vi "WriteTDMSTest1.vi"() -> ()   [LabVIEW 2016]
panel:
  out "Experiment Description 2":T1={"Sample Description"={"sample name"="SA01234.A", "device"="SA01234.A.20180713", "user"="patrick", "project"="graphene", "description"="sketch SET", "sample GUID"="3EAEE46B-2F5E-4712-8AE3-C241FD138412"}, "Experiment Description"={"folder name"="G:\\data\\graphene\\SA01234.A.20180713", "user description"="sweep Vsg as a function of B", "experiment GUID"="30E3DD13-C39C-4090-BB9A-3764BBD20948", "loop info (?)"=""}, "Krohn-Hite"={"Krohn-Hite Channel Array"=[{"channel"="Channel 1", "input config"="Differential", "gain"=100, "shunt resistor"=50, "input coupling"="", "filter"=""}, {"channel"="Channel 2", "input config"="Differential", "gain"=10, "shunt resistor"=50, "input coupling"="", "filter"=""}, {"channel"="Channel 3", "input config"="SE+ (-gnd)", "gain"=10, "shunt resistor"=0, "input coupling"="", "filter"=""}, {"channel"="Channel 4", "input config"="SE+ (-gnd)", "gain"=10, "shunt resistor"=0, "input coupling"="", "filter"=""}, {"channel"="Channel 5", "input config"="SE+ (-gnd)", "gain"=10, "shunt resistor"=0, "input coupling"="", "filter"=""}]}, "Lockin"={"Lockin AO"={"Lockin AO Channel Array"=[{"name"="0", "amplitude"=0.0, "DC offset"=0.0, "frequency"=13.0, "phase"=0.0, "function"="Sine"}, {"name"="1", "amplitude"=0.0, "DC offset"=0.0, "frequency"=13.0, "phase"=0.0, "function"="Sine"}, {"name"="2", "amplitude"=0.0, "DC offset"=0.0, "frequency"=13.0, "phase"=0.0, "function"="Sine"}, {"name"="3", "amplitude"=0.0, "DC offset"=0.0, "frequency"=13.0, "phase"=0.0, "function"="Sine"}, {"name"="4", "amplitude"=0.0, "DC offset"=0.0, "frequency"=13.0, "phase"=0.0, "function"="Sine"}, {"name"="5", "amplitude"=0.0, "DC offset"=0.0, "frequency"=13.0, "phase"=0.0, "function"="Sine"}, {"name"="6", "amplitude"=0.0, "DC offset"=0.0, "frequency"=13.0, "phase"=0.0, "function"="Sine"}, {"name"="7", "amplitude"=0.0, "DC offset"=0.0, "frequency"=13.0, "phase"=0.0, "function"="Sine"}]}, "Lockin AI"={"Lockin AI Array"=[{"KH Channel"="Channel 1", "AI Channel"="0"}, {"KH Channel"="Channel 2", "AI Channel"="1"}, {"KH Channel"="Channel 3", "AI Channel"="2"}, {"KH Channel"="Channel 4", "AI Channel"="3"}, {"KH Channel"="Channel 5", "AI Channel"="4"}]}, "Lockin REF"={"Lockin REF Array"=[{"frequency"=13.0, "phase"=0.0}]}}}
  out "date/time string":string="2018-10-02--21-17-20"
  out "current time":timestamp=timestamp(3621359841.3756013 s since 1904-01-01)
  in  "file path":path=path "C:/Users/Patrick/Desktop/TEST/TEST.tdms"
  in  "stop":bool
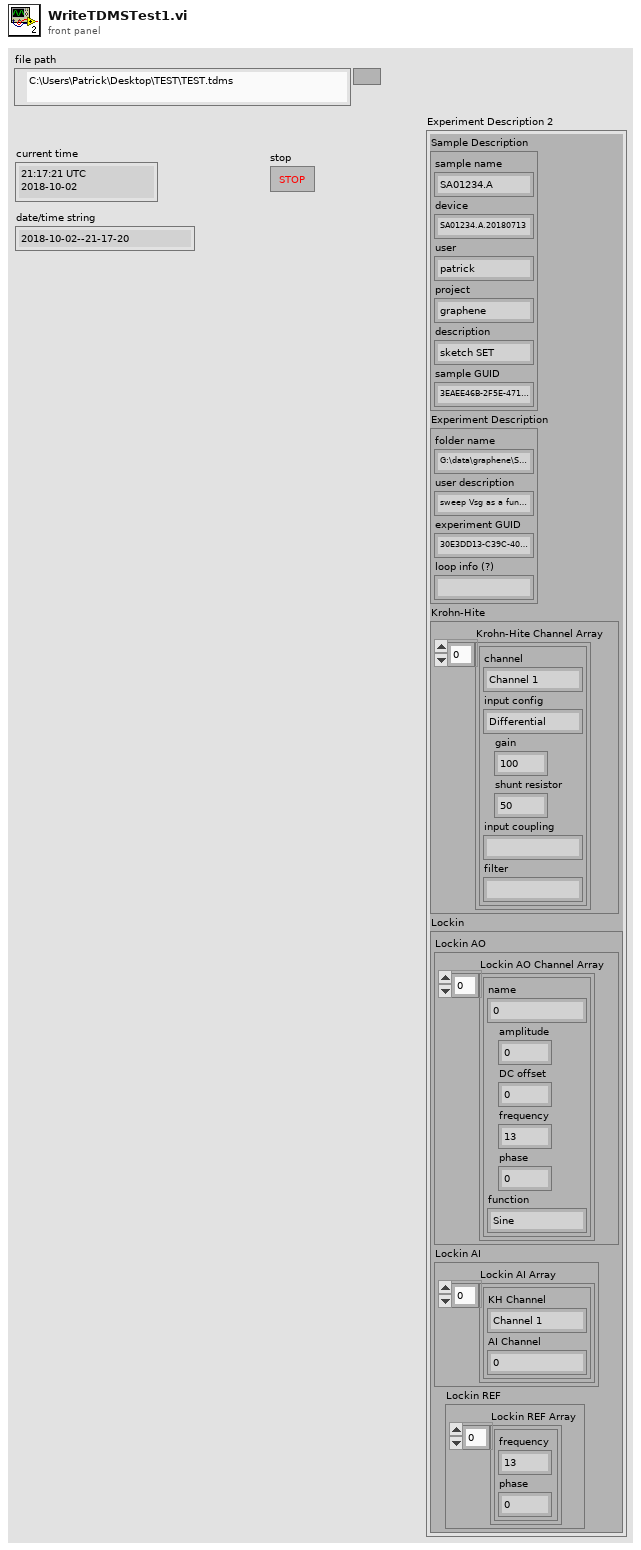
[diagram p1: front panel]
types:
  T1 = cluster{"Sample Description":cluster{"sample name":string, "device":string, "user":string, "project":string, "description":string, "sample GUID":string}, "Experiment Description":cluster{"folder name":string, "user description":string, "experiment GUID":string, "loop info (?)":string}, "Krohn-Hite":cluster{"Krohn-Hite Channel Array":cluster{"channel":string, "input config":string, "gain":i32, "shunt resistor":i32, "input coupling":string, "filter":string}[]}, "Lockin":cluster{"Lockin AO":cluster{"Lockin AO Channel Array":cluster{"name":string, "amplitude":dbl, "DC offset":dbl, "frequency":dbl, "phase":dbl, "function":string}[]}, "Lockin AI":cluster{"Lockin AI Array":cluster{"KH Channel":string, "AI Channel":string}[]}, "Lockin REF":cluster{"Lockin REF Array":cluster{"frequency":dbl, "phase":dbl}[]}}}
  T2 = enum16{"open", "open or create", "create or replace", "create", "open (read-only)"}
  T3 = cluster{"Sample Description":cluster{"name":string, "device":string, "user":string, "project":string, "description":string, "sample GUID":string}, "Experiment Description":cluster{"folder name":string, "user description":string, "experiment GUID":string, "loop info (?)":string}, "Krohn-Hite":cluster{"Krohn-Hite Channel Array":cluster{"channel":string, "input config":string, "gain":i32, "shunt resistor":i32, "input coupling":string, "filter":string}[]}, "Lockin":cluster{"Lockin AO":cluster{"Lockin AO Channel Array":cluster{"name":string, "amplitude":dbl, "DC offset":dbl, "frequency":dbl, "phase":dbl, "function":string}[]}, "Lockin AI":cluster{"Lockin AI Array":cluster{"KH Channel":string, "AI Channel":string}[]}, "Lockin REF":cluster{"Lockin REF Array":cluster{"frequency":dbl, "phase":dbl}[]}}}
  T4 = cluster{"name":string, "device":string, "user":string, "project":string, "description":string, "sample GUID":string}
  T5 = cluster{"folder name":string, "user description":string, "experiment GUID":string, "loop info (?)":string}
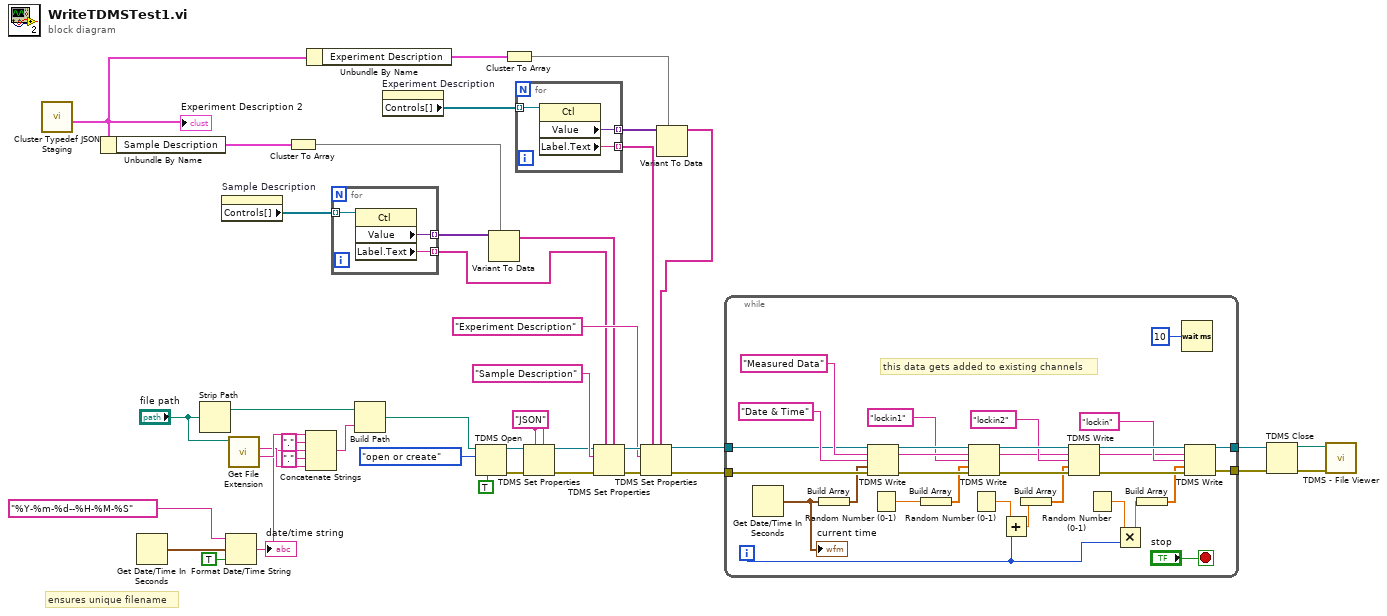
[diagram p0: block diagram]
diagram:
  w6 = "JSON"
  # "ensures unique filename"
  n1 = call "Cluster Typedef JSON Staging.vi"() -> ("Experiment Description 2"=w19:T3)  [unwired: 9 in, 2 out]
  "Experiment Description 2" <- w19
  n2 = Unbundle By Name(w19) -> ("Sample Description"=w4:T4)
  n3 = Get Date/Time In Seconds() -> (seconds since 1Jan1904=w39:timestamp)
  n4 = Strip Path(path="file path") -> (stripped path=w26:path)  [unwired: 1 out]
  n5 = property on="Sample Description" class="Clust (strict)"() -> ("Controls[]"=w42:refnum<vi>[])  [unwired: 2 in, 2 out]
  n6 = Format Date/Time String(time format string (%c)="%Y-%m-%d--%H-%M-%S", seconds (now)=w39, UTC format=TRUE) -> (date/time string=w35:string)
  "date/time string" <- w35
  n7 = call <vilib>:"Get File Extension.vi"("file"="file path") -> ("filename without extension"=w37:string, "lowercase file extension"=w36:string)  [unwired: 6 in, 3 out]
  n8 = Cluster To Array(cluster=w4) -> (array=w5:string[])
  n9 = Concatenate Strings(w37, "." ("string"), w35, "." ("string"), w36) -> (w25:string)
  n10 = Unbundle By Name(w19) -> ("Experiment Description"=w23:T5)
  n11 = for {
    tunnel: w42 -> [w45] mode=indexing
    tunnel: [w44] -> w41 mode=indexing
    tunnel: [w43] -> w2 mode=indexing
    n12 = property class="Ctl"(reference=w45) -> ("Value"=w44:variant, "Label.Text"=w43:string)  [unwired: 1 in, 2 out]
  }
  n13 = Build Path(base path=w26, name or relative path=w25) -> (appended path=w24:path)
  n14 = property on="Experiment Description" class="Clust (strict)"() -> ("Controls[]"=w20:refnum<vi>[])  [unwired: 2 in, 2 out]
  n15 = TDMS Open(6:TRUE ("disable buffering? (T)"), 10:T2."open or create" ("operation (0:open)"), 11:w24) -> (0:w12:errorcluster, 3:w11:refnum<k34>)  [unwired: 4 in]
  n16 = Variant To Data(type=w5, Variant=w41) -> (data=w3:string[])  [unwired: 1 in, 1 out]
  n17 = Cluster To Array(cluster=w23) -> (array=w22:string[])
  n18 = for {
    tunnel: w20 -> [w48] mode=indexing
    tunnel: [w47] -> w21 mode=indexing
    tunnel: [w46] -> w16 mode=indexing
    n19 = property class="Ctl"(reference=w48) -> ("Value"=w47:variant, "Label.Text"=w46:string)  [unwired: 1 in, 2 out]
  }
  n20 = TDMS Set Properties(5:w6, 7:w6, 8:w12, 11:w11) -> (0:w9:errorcluster, 3:w10:refnum<k34>)  [unwired: 2 in, 2 out]
  n21 = TDMS Set Properties(5:w3, 7:w2, 8:w9, 10:"Sample Description" ("group name"), 11:w10) -> (0:w18:errorcluster, 3:w17:refnum<k34>)  [unwired: 1 in, 2 out]
  n22 = Variant To Data(type=w22, Variant=w21) -> (data=w1:string[])  [unwired: 1 in, 1 out]
  n23 = TDMS Set Properties(5:w1, 7:w16, 8:w18, 10:"Experiment Description" ("group name"), 11:w17) -> (0:w8:errorcluster, 3:w7:refnum<k34>)  [unwired: 1 in, 2 out]
  n24 = while {
    tunnel: w8 -> [w76]
    tunnel: [w57] -> w28
    tunnel: [w56] -> w27
    tunnel: w7 -> [w50]
    i -> [w49]
    stop <- "stop" stop-if-true
    # "this data gets added to existing channels"
    n25 = Get Date/Time In Seconds() -> (seconds since 1Jan1904=w55:timestamp)
    "current time" <- w55
    n26 = Build Array(w55) -> (w74:timestamp[])
    n27 = TDMS Write(0:w50, 5:"Measured Data" ("group name in (Untitled)"), 7:"Date & Time", 9:w74, 11:w76) -> (4:w73:refnum<k34>, 6:w71:string, 15:w72:errorcluster)  [unwired: 1 in, 1 out]
    n28 = Random Number (0-1)() -> (number: 0 to 1=w69:dbl)
    n29 = Build Array(w69) -> (w68:dbl[])
    n30 = TDMS Write(0:w73, 5:w71, 7:"lockin1", 9:w68, 11:w72) -> (4:w67:refnum<k34>, 6:w62:string, 15:w66:errorcluster)  [unwired: 1 in, 1 out]
    n31 = Random Number (0-1)() -> (number: 0 to 1=w52:dbl)
    n32 = Add(x=w52, y=w49) -> (x+y=w51:dbl)
    n33 = Build Array(w51) -> (w61:dbl[])
    n34 = TDMS Write(0:w67, 5:w62, 7:"lockin2", 9:w61, 11:w66) -> (4:w65:refnum<k34>, 6:w58:string, 15:w64:errorcluster)  [unwired: 1 in, 1 out]
    n35 = Random Number (0-1)() -> (number: 0 to 1=w54:dbl)
    n36 = Multiply(x=w54, y=w49) -> (x*y=w53:dbl)
    n37 = Build Array(w53) -> (w60:dbl[])
    n38 = Wait (ms)(milliseconds to wait=u32 10) -> ()  [unwired: 1 out]
    n39 = TDMS Write(0:w65, 5:w58, 7:"lockin", 9:w60, 11:w64) -> (4:w57:refnum<k34>, 15:w56:errorcluster)  [unwired: 1 in, 2 out]
  }
  n40 = TDMS Close(8:w27, 11:w28) -> (0:w30:errorcluster, 3:w29:path)
  n41 = call <vilib>:"TDMS - File Viewer.vi"("error in (no error)"=w30, "file path"=w29) -> ()  [unwired: 4 in, 2 out]
